vi "decimate-value_multiple_axis.vi"(7 "type":T1, 8 "error in (no error)":errorcluster, 9 "interval":dbl format="%#_13g", 10 "y_axis in":dbl[][](array[numeric]), 11 "x_axis in":dbl[](array[numeric])) -> (0 "error out":errorcluster, 2 "y_axis out":dbl[][](array[numeric]), 3 "x_axis out":dbl[](array[numeric]))   [LabVIEW 2015, in "lv-graph.lvlib"]
doc: "This VI will decimate a given dataset, following the rule that you can display, at most two points per pixel per plot. If the number of points exceeds the number of pixels (wired from height_width). For decimation, it'll group equal sets of points (except the last set) for data representation. As configured, the way the points are represented can be configured as follows: (1) average: this will get the mean of the points per group (2) min_max will average the min/max values for the group (3) max: will return the max value, (4) min: will return the min value, (5) first will return the first value and (6) last will return the last value."
uses:
  lv-graph.lvlib
  _controls/decimation_type.ctl
  <vilib>/Analysis/baseanly.llb/Mean (DBL).vi
  <vilib>/Analysis/NI_AALBase.lvlib
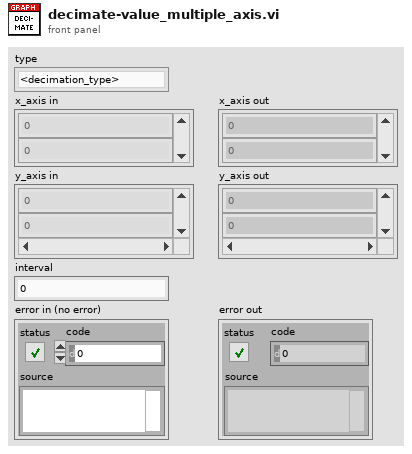
[diagram p1: front panel]
types:
  T1 = typedef "lv-graph.lvlib/decimation_type.ctl" = enum16{"<decimation_type>", "average", "min_max", "max", "min", "first", "last"}
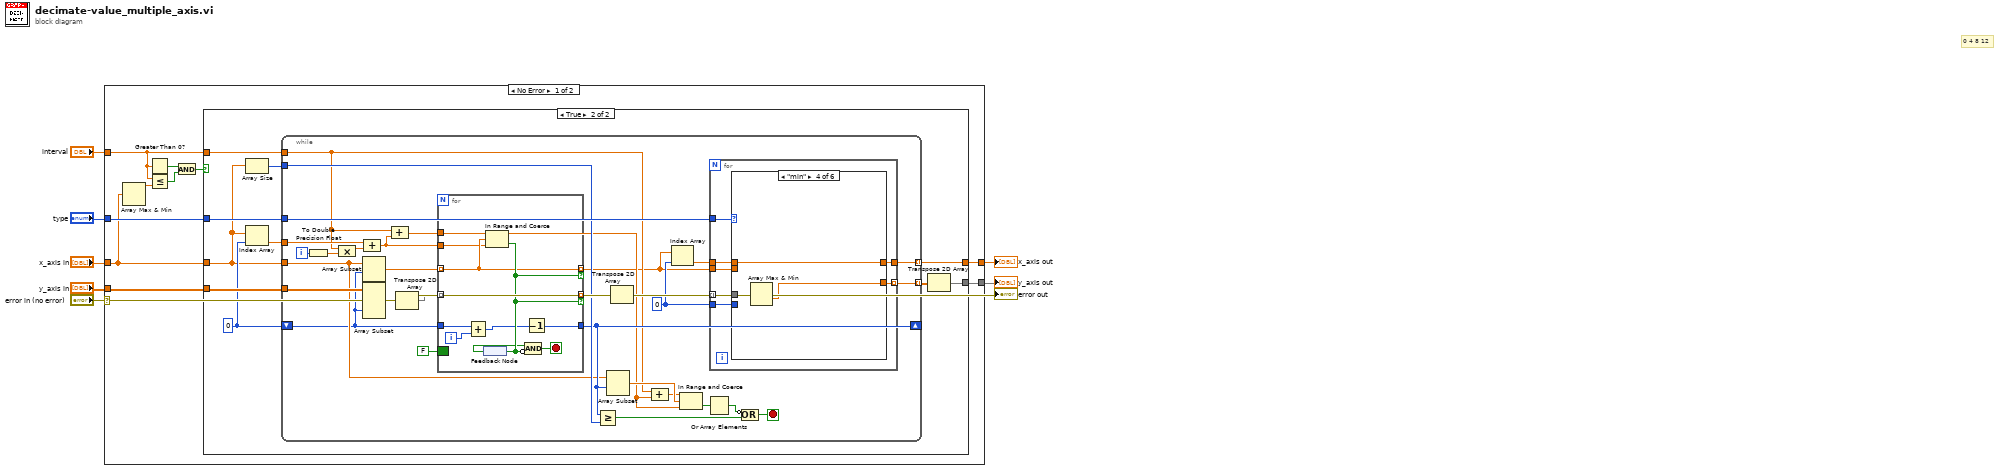
[diagram p0: block diagram]
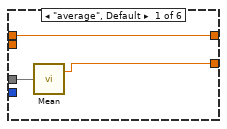
[diagram p3: hidden frame]
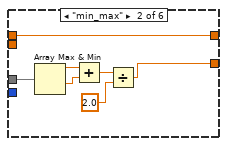
[diagram p4: hidden frame]
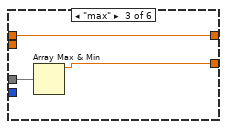
[diagram p5: hidden frame]
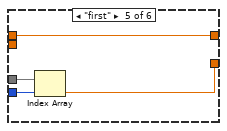
[diagram p6: hidden frame]
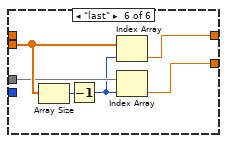
[diagram p7: hidden frame]
diagram:
  # "0 4 8 12"
  n1 = case shown="No Error" "error in (no error)" {
    tunnel: "x_axis in" -> [w8 _]
    tunnel: "y_axis in" -> [w13 _]
    tunnel: "type" -> [w17 _]
    tunnel: [w16 _] -> w2
    tunnel: [w15 _] -> w1
    tunnel: "interval" -> [w11 _]
    frame No Error {
      n2 = Array Max & Min(array=w8) -> (max value=w12:dbl)  [unwired: 3 out]
      n3 = Greater Than 0?(x=w11) -> (x > 0?=w14:bool)
      n4 = Less Or Equal?(x=w11, y=w12) -> (x <= y?=w9:bool)
      n5 = And(x=w14, y=w9) -> (x .and. y?=w10:bool)
      n6 = case shown="True" w10 {
        tunnel: w8 -> [w19 w23]
        tunnel: w13 -> [w18 w27]
        tunnel: w17 -> [_ w29]
        tunnel: [w19 w28] -> w16
        tunnel: [w18 w20] -> w15
        tunnel: w11 -> [_ w26]
        frame False {
        }
        frame True {
          w24 = 0
          n7 = Array Size(array=w23) -> (size(s)=w22:i32)
          n8 = Index Array(array=w23, index=w24) -> (element=w25:dbl)
          n9 = while {
            tunnel: w29 -> [w58]
            tunnel: [w35] -> w21 mode=indexing
            tunnel: [w59] -> w28 mode=indexing
            tunnel: w23 -> [w48]
            tunnel: w27 -> [w53]
            shift-right: [w52] -> _
            shift-left: w24 -> [w34]
            tunnel: w26 -> [w40]
            tunnel: w22 -> [w54]
            tunnel: w25 -> [w44]
            i -> [w41]
            stop <- w38 stop-if-true
            w37 = 0 ("index")
            n10 = To Double Precision Float(number=w41) -> (double precision float=w47:dbl)
            n11 = Compound Arithmetic op=MULTIPLY(w40, w47) -> (w45:dbl)
            n12 = Array Subset(array=w48, index=w34) -> (w56:dbl[])  [unwired: 1 in]
            n13 = Array Subset(array=w53, index (col)=w34) -> (w55:dbl[][])  [unwired: 3 in]
            n14 = Compound Arithmetic op=ADD(w44, w45) -> (w43:dbl)
            n15 = Compound Arithmetic op=ADD(w40, w43) -> (w42:dbl)
            n16 = Transpose 2D Array(2D array=w55) -> (transposed array=w31:dbl[][])
            n17 = for {
              tunnel: w34 -> [w103]
              tunnel: [w93] -> w52
              tunnel: w56 -> [w98] mode=indexing
              tunnel: w31 -> [w97] mode=indexing
              tunnel: [w98] -> w33 mode=indexing if=w101
              tunnel: [w97] -> w57 mode=indexing if=w101
              tunnel: w43 -> [w95]
              tunnel: w42 -> [w94]
              border: FALSE -> [_]
              i -> [w102]
              stop <- w96 stop-if-true
              n18 = Add(x=w103, y=w102) -> (x+y=w99:i32)
              n19 = feedback #1() -> (w100:bool)
              n20 = In Range and Coerce(upper limit=w94, x=w98, lower limit=w95) -> (In Range?=w101:bool)  [unwired: 1 out]
              n21 = feedback-in #1(w101) -> ()
              n22 = Decrement(x=w99) -> (x-1=w93:i32)
              n23 = Compound Arithmetic op=AND(w100, invert w101) -> (w96:bool)
            }
            n24 = Greater Or Equal?(x=w52, y=w54) -> (x >= y?=w39:bool)
            n25 = Array Subset(array=w48, index=w52) -> (w51:dbl[])  [unwired: 1 in]
            n26 = Transpose 2D Array(2D array=w57) -> (transposed array=w30:dbl[][])
            n27 = Compound Arithmetic op=ADD(w40, w42) -> (w46:dbl)
            n28 = Index Array(array=w33, index=w37) -> (element=w36:dbl)
            n29 = In Range and Coerce(upper limit=w46, x=w51, lower limit=w42) -> (In Range?=w50:bool[])  [unwired: 1 out]
            n30 = Or Array Elements(Boolean array=w50) -> (logical OR=w49:bool)
            n31 = for {
              tunnel: [w66] -> w35 mode=indexing
              tunnel: [w65] -> w59
              tunnel: w58 -> [w64]
              tunnel: w33 -> [w63]
              tunnel: w37 -> [w62]
              tunnel: w36 -> [w61]
              tunnel: w30 -> [w60] mode=indexing
              n32 = case shown="\"min\"" w64 {
                tunnel: w63 -> [_ _ _ _ _ w90]
                tunnel: w60 -> [w69 w76 w79 w82 w86 w88]
                tunnel: [w68 w75 w78 w81 w85 w91] -> w66
                tunnel: [w67 w70 w77 w80 w83 w92] -> w65
                tunnel: w62 -> [_ _ _ _ w84 _]
                tunnel: w61 -> [w67 w70 w77 w80 w83 _]
                frame "average", Default {
                  n33 = call-poly <vilib>:"Mean.vi"("X"=w69) -> ("mean"=w68:dbl)  [unwired: 1 out]
                }
                frame "min_max" {
                  n34 = Array Max & Min(array=w76) -> (max value=w74:dbl, min value=w73:dbl)  [unwired: 2 out]
                  n35 = Add(x=w74, y=w73) -> (x+y=w72:dbl)
                  n36 = Divide(x=w72, y=2.0) -> (x/y=w75:dbl)
                }
                frame "max" {
                  n37 = Array Max & Min(array=w79) -> (max value=w78:dbl)  [unwired: 3 out]
                }
                frame "min" {
                  n38 = Array Max & Min(array=w82) -> (min value=w81:dbl)  [unwired: 3 out]
                }
                frame "first" {
                  n39 = Index Array(array=w86, index=w84) -> (element=w85:dbl)
                }
                frame "last" {
                  n40 = Array Size(array=w90) -> (size(s)=w89:i32)
                  n41 = Decrement(x=w89) -> (x-1=w87:i32)
                  n42 = Index Array(array=w90, index=w87) -> (element=w92:dbl)
                  n43 = Index Array(array=w88, index=w87) -> (element=w91:dbl)
                }
              }
            }
            n44 = Compound Arithmetic op=OR(invert w49, w39) -> (w38:bool)
          }
          n45 = Transpose 2D Array(2D array=w21) -> (transposed array=w20:dbl[][])
        }
      }
    }
    frame Error {
    }
  }
  "x_axis out" <- w2
  "y_axis out" <- w1
  "error out" <- "error in (no error)"
